vi "CustomCollector.vi"(6 "Reset":bool, 8 "error in (no error)":errorcluster, 9 "Enable":bool=TRUE, 10 "Size":u32=600, 11 "Signals":dynamicdata(graph)) -> (0 "error out":errorcluster, 2 "Collected Signals":dynamicdata(graph))   [LabVIEW 2014]
doc: "Collects input signals and returns the most recent data, up to the specified maximum number of samples per channel. When you call this Express VI repeatedly and the Express VI reaches the maximum number of samples per channel, the Express VI discards the oldest data and adds the newest data to the collected samples.\n--------------------\n\nThis Express VI is configured as follows:\n\nNumber of Points to Collect: 600"
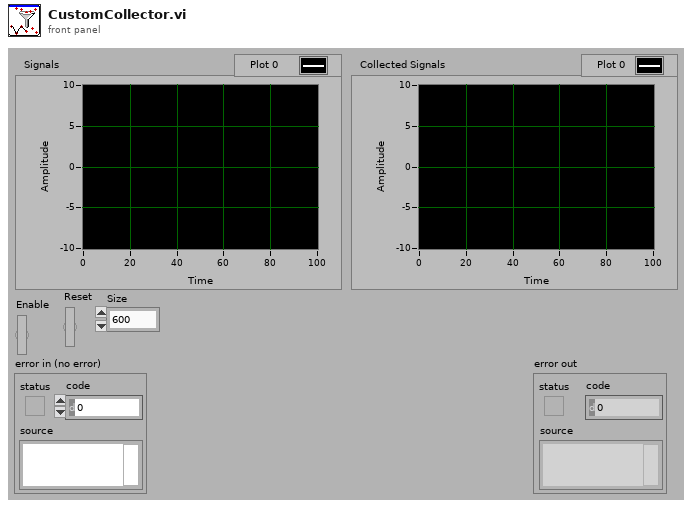
[diagram p1: front panel]
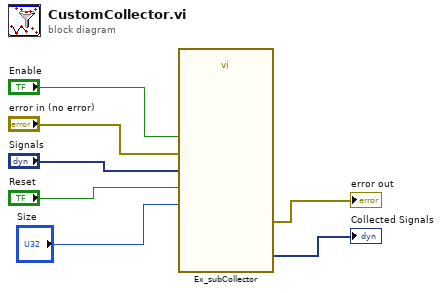
[diagram p0: block diagram]
diagram:
  n1 = call <vilib>:"Ex_subCollector.vi"("Input"="Signals", "Reset"="Reset", "Enable"="Enable", "error in (no error)"="error in (no error)", "Size"="Size") -> ("Waveform Output"=→"Collected Signals":dynamicdata, "error out"=→"error out":errorcluster)  [unwired: 12 in, 1 out]
